vi "Set Limit.vi"(8 "Error In":errorcluster, 10 "Limit":u32, 11 "ByteBuffer In":refnum<class "ByteBuffer.lvclass">) -> (0 "Error Out":errorcluster, 3 "ByteBuffer Out":refnum<class "ByteBuffer.lvclass">)   [LabVIEW 2015, in "ByteBuffer.lvclass"]
doc: "Sets this buffer's limit. If the position is larger than the new limit then it is set to the new limit. If the mark is defined and larger than the new limit then it is discarded.\n\nParameters:\n+ Limit - The new limit value, must be non-negative and no larger than this buffer's capacity.\n\nReturns:\nThis buffer.\n\nThrows:\n+ IllegalArgumentException - If the preconditions on new limit do not hold."
uses:
  ByteBuffer.lvclass
  ByteBuffer.lvclass/ByteBuffer.ctl
  <vilib>/Utility/error.llb/Error Cluster From Error Code.vi
  <vilib>/ErrorRing/Error Ring.xnode
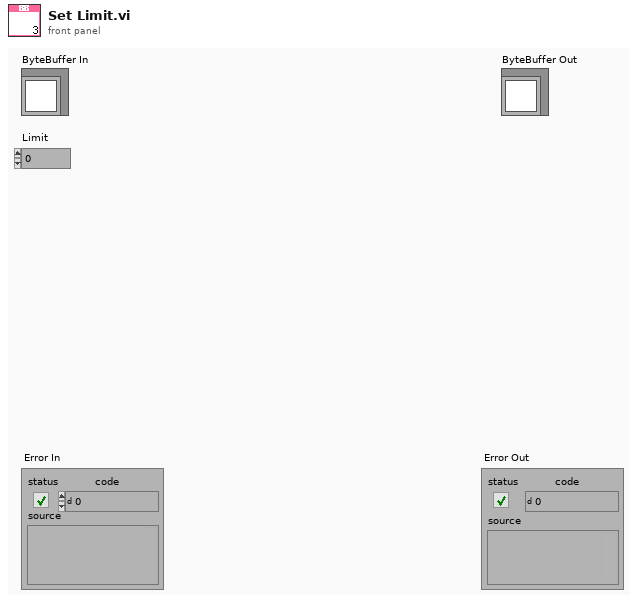
[diagram p1: front panel]
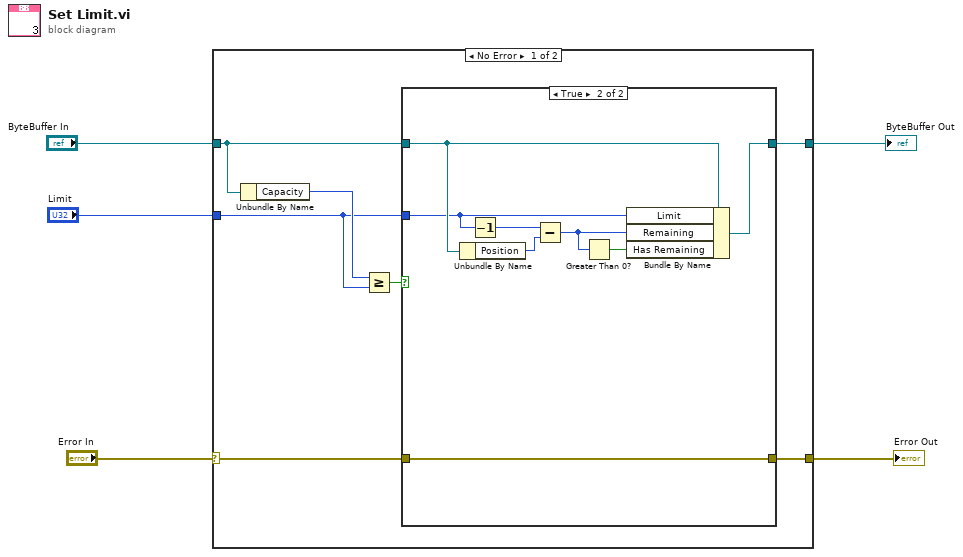
[diagram p0: block diagram]
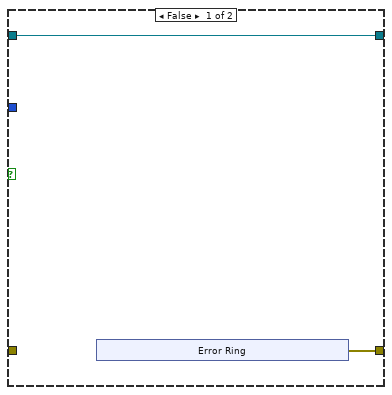
[diagram p2: hidden frame]
diagram:
  n1 = case shown="No Error" "Error In" {
    selector: "Error In" -> [w9 w29]
    tunnel: [w6 w29] -> w4
    tunnel: "ByteBuffer In" -> [w11 w28]
    tunnel: "Limit" -> [w7 _]
    tunnel: [w12 w28] -> w1
    frame No Error {
      n2 = Unbundle By Name(w11) -> ("Capacity"=w10:u32)
      n3 = Greater Or Equal?(x=w10, y=w7) -> (x >= y?=w8:bool)
      n4 = case shown="True" w8 {
        tunnel: [w14 w27] -> w12
        tunnel: w11 -> [w14 w25]
        tunnel: w9 -> [_ w26]
        tunnel: w7 -> [_ w24]
        tunnel: [w13 w26] -> w6
        frame False {
          n5 = xnode "Error Ring"() -> ("error out"=w13:errorcluster)
        }
        frame True {
          n6 = Unbundle By Name(w25) -> ("Position"=w23:u32)
          n7 = Decrement(x=w24) -> (x-1=w22:u32)
          n8 = Subtract(x=w22, y=w23) -> (x-y=w20:u32)
          n9 = Greater Than 0?(x=w20) -> (x > 0?=w21:bool)
          n10 = Bundle By Name(cluster=w25, "Limit"=w24, "Remaining"=w20, "Has Remaining"=w21) -> (w27:refnum<class "ByteBuffer.lvclass">)
        }
      }
    }
    frame Error {
    }
  }
  "Error Out" <- w4
  "ByteBuffer Out" <- w1
